vi "PM5000_random.vi"(1 "Variacion Frecuencia":sgl=0.1, 2 "Variacion Voltaje":sgl=5.0, 3 "Señal":sgl=230.0, 4 "Signal In":T1) -> (0 "Signal Out":sgl)   [LabVIEW 2018]
uses:
  Controls/Action_demo.ctl
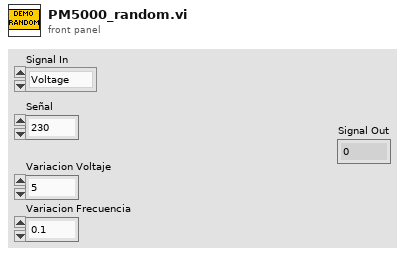
[diagram p1: front panel]
types:
  T1 = typedef "Action_demo.ctl" = enum16{"Voltage", "Polar", "Frecuency", "Current", "Power", "THD"}
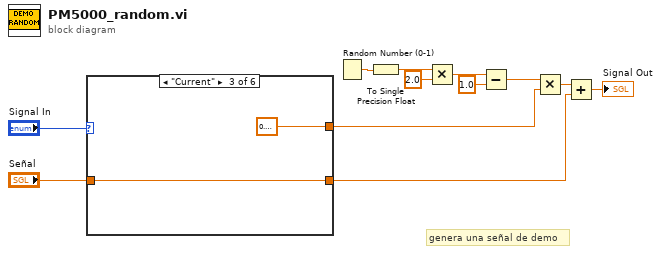
[diagram p0: block diagram]
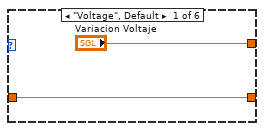
[diagram p2: hidden frame]
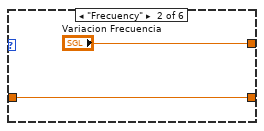
[diagram p3: hidden frame]
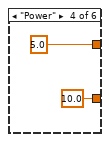
[diagram p4: hidden frame]
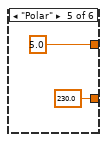
[diagram p5: hidden frame]
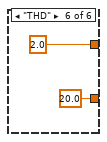
[diagram p6: hidden frame]
diagram:
  # "genera una señal de demo"
  n1 = case shown="\"Current\"" "Signal In" {
    tunnel: ["Variacion Voltaje" "Variacion Frecuencia" sgl 0.1 ("y") sgl 5.0 ("y") sgl 5.0 ("y") sgl 2.0 ("y")] -> w6
    tunnel: [w14 w16 w17 sgl 10.0 ("THD") sgl 230.0 ("THD") sgl 20.0 ("THD")] -> w1
    tunnel: "Señal" -> [w14 w16 w17 _ _ _]
    frame "Voltage", Default {
    }
    frame "Frecuency" {
    }
    frame "Current" {
    }
    frame "Power" {
    }
    frame "Polar" {
    }
    frame "THD" {
    }
  }
  n2 = Random Number (0-1)() -> (number: 0 to 1=w9:dbl)
  n3 = To Single Precision Float(number=w9) -> (single precision float=w8:sgl)
  n4 = Multiply(x=w8, y=sgl 2.0) -> (x*y=w11:sgl)
  n5 = Subtract(x=w11, y=sgl 1.0) -> (x-y=w7:sgl)
  n6 = Multiply(x=w7, y=w6) -> (x*y=w5:sgl)
  n7 = Add(x=w5, y=w1) -> (x+y=→"Signal Out":sgl)
